vi "Stop Core.vi"(10 "final error code":i32, 11 "Generic Card in":refnum<class "Generic Card.lvclass">) -> (3 "Generic Card out":refnum<class "Generic Card.lvclass">)   [LabVIEW 2013, in "Generic Instrument.lvlib" / "Generic Card.lvclass"]
doc: "(<B>Filename</B>: Actor Framework.lvlib:Actor.lvclass:Stop Core.vi)\n\nDefines what the actor does before it stops. Use the <B>final error code</B> input to determine whether the actor shut down in response to an error.\n\nBy default, this method does nothing. A descendant class may override it to define behavior, such as shutting down any processes the actor initiated in its override of the Actor Core method."
uses:
  Generic Card.lvclass
  WT1600 Card/Observer Pattern Actor Template/Observer/Observer.lvclass
  <vilib>/ActorFramework/Stop Msg/Stop Msg.lvclass
  <vilib>/ActorFramework/Actor/Actor.lvclass
  Universal Power Meter/Universal Power Meter class/Universal Power Meter.lvclass
  Generic Instrument.lvclass
panel:
  in  "error in (no error)":errorcluster
  out "error out":errorcluster
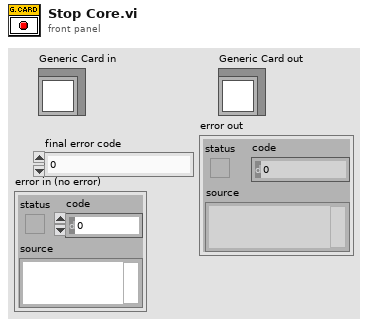
[diagram p1: front panel]
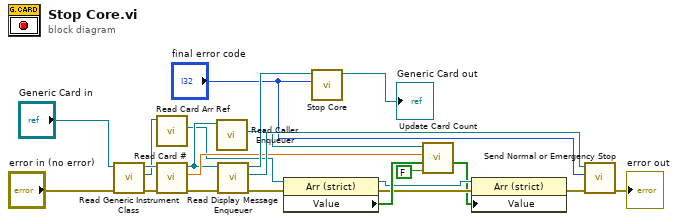
[diagram p0: block diagram]
diagram:
  n1 = call "Read Generic Instrument Class.vi"("error in (no error)"="error in (no error)", "Generic Card in"="Generic Card in") -> ("error out"=w12:errorcluster, "Generic Instrument.lvlib:Generic Instrument.lvclass"=w11:refnum<class "Generic Instrument.lvclass">, "Generic Card out"=w13:refnum<class "Generic Card.lvclass">)  [unwired: 7 in]
  n2 = call-dynamic "Read Card Arr Ref.vi"("Generic Instrument in"=w11) -> ("Card Arr Ref"=w10:refnum<vi>)  [unwired: 8 in, 2 out]
  n3 = call "Read Card #.vi"("error in (no error)"=w12, "Generic Card in"=w13) -> ("error out"=w15:errorcluster, "Card #"=w18:dbl, "Generic Card out"=w16:refnum<class "Generic Card.lvclass">)  [unwired: 7 in]
  n4 = call <vilib>:"Read Caller Enqueuer.vi"("Actor"=w16) -> ("Caller Enqueuer"=w17:refnum<class "Message Enqueuer.lvclass">)  [unwired: 10 in]
  n5 = call "Read Display Message Enqueuer.vi"("error in (no error)"=w15, "Generic Card in"=w16) -> ("error out"=w5:errorcluster, "Actor Framework.lvlib:Message Enqueuer"=w20:refnum<class "Message Enqueuer.lvclass">, "Generic Card out"=w21:refnum<class "Generic Card.lvclass">)  [unwired: 7 in]
  n6 = property class="Arr (strict)"(reference=w10, error in=w5) -> (reference out=w8:refnum<vi>, error out=w7:errorcluster, "Value"=w9:bool[])
  n7 = call-parent "Stop Core.vi"("final error code"="final error code", "Actor in"=w21) -> ("Actor out"=→"Generic Card out":refnum<class "Generic Card.lvclass">)  [unwired: 9 in]
  n8 = call "Update Card Count.vi"("new element/subarray"=FALSE, "Card Array in"=w9, "# in"=w18, "Message Enqueuer"=w17) -> ("Card Array Out"=w6:bool[])  [unwired: 6 in, 1 out]
  n9 = property class="Arr (strict)"(reference=w8, error in=w7, "Value"=w6) -> (error out=w4:errorcluster)  [unwired: 1 out]
  n10 = call <vilib>:"Send Normal or Emergency Stop.vi"("error in (no error)"=w4, "final error code"="final error code", "Message Enqueuer"=w20) -> ("error out"=→"error out":errorcluster)  [unwired: 8 in]
